vi "StripQuotesOnString.vi"(10 "String":string) -> (2 "Unquoted String":string)   [LabVIEW 2021, in "Bananas.lvlib" / "BananaPeel.lvclass"]
uses:
  BananaPeel.Project/Project.lvclass/Project.ctl
  BananaPeel.lvclass
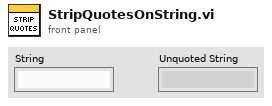
[diagram p1: front panel]
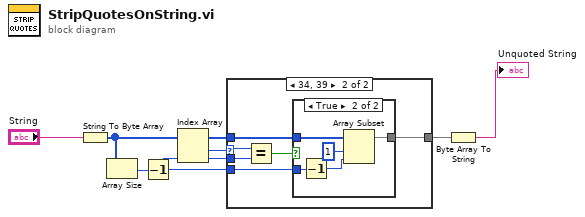
[diagram p0: block diagram]
diagram:
  n1 = String To Byte Array(string="String") -> (unsigned byte array=w5:u8[])
  n2 = Array Size(array=w5) -> (size(s)=w2:i32)
  n3 = Decrement(x=w2) -> (x-1=w8:i32)
  n4 = Index Array(array=w5, index #2=w8) -> (element #1=w1:u8, element #2=w3:u8)  [unwired: 1 in]
  n5 = case shown="34, 39" w1 {
    selector: w1 -> [_ w15]
    tunnel: w3 -> [_ w14]
    tunnel: w5 -> [w9 w13]
    tunnel: [w9 w11] -> w6
    tunnel: w8 -> [_ w10]
    frame Default {
    }
    frame 34, 39 {
      n6 = Equal?(x=w15, y=w14) -> (x = y?=w12:bool)
      n7 = case shown="True" w12 {
        tunnel: w13 -> [w16 w21]
        tunnel: [w16 w20] -> w11
        tunnel: w10 -> [_ w18]
        frame False {
        }
        frame True {
          n8 = Decrement(x=w18) -> (x-1=w17:i32)
          n9 = Array Subset(array=w21, index=1, length=w17) -> (w20:u8[])
        }
      }
    }
  }
  n10 = Byte Array To String(unsigned byte array=w6) -> (string=→"Unquoted String":string)
